vi "average position.vi"(1 "num lights":dbl, 2 "XYZ out":T1(array[cluster])) -> (0 "Lights pos":dbl[][](array[numeric]))   [LabVIEW 2011]
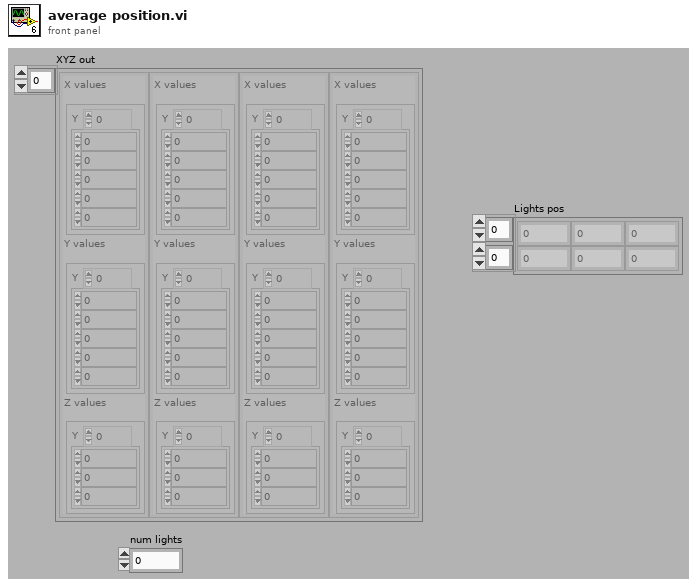
[diagram p1: front panel]
types:
  T1 = cluster{"X values":waveform(dbl), "Y values":waveform(dbl), "Z values":waveform(dbl)}[]
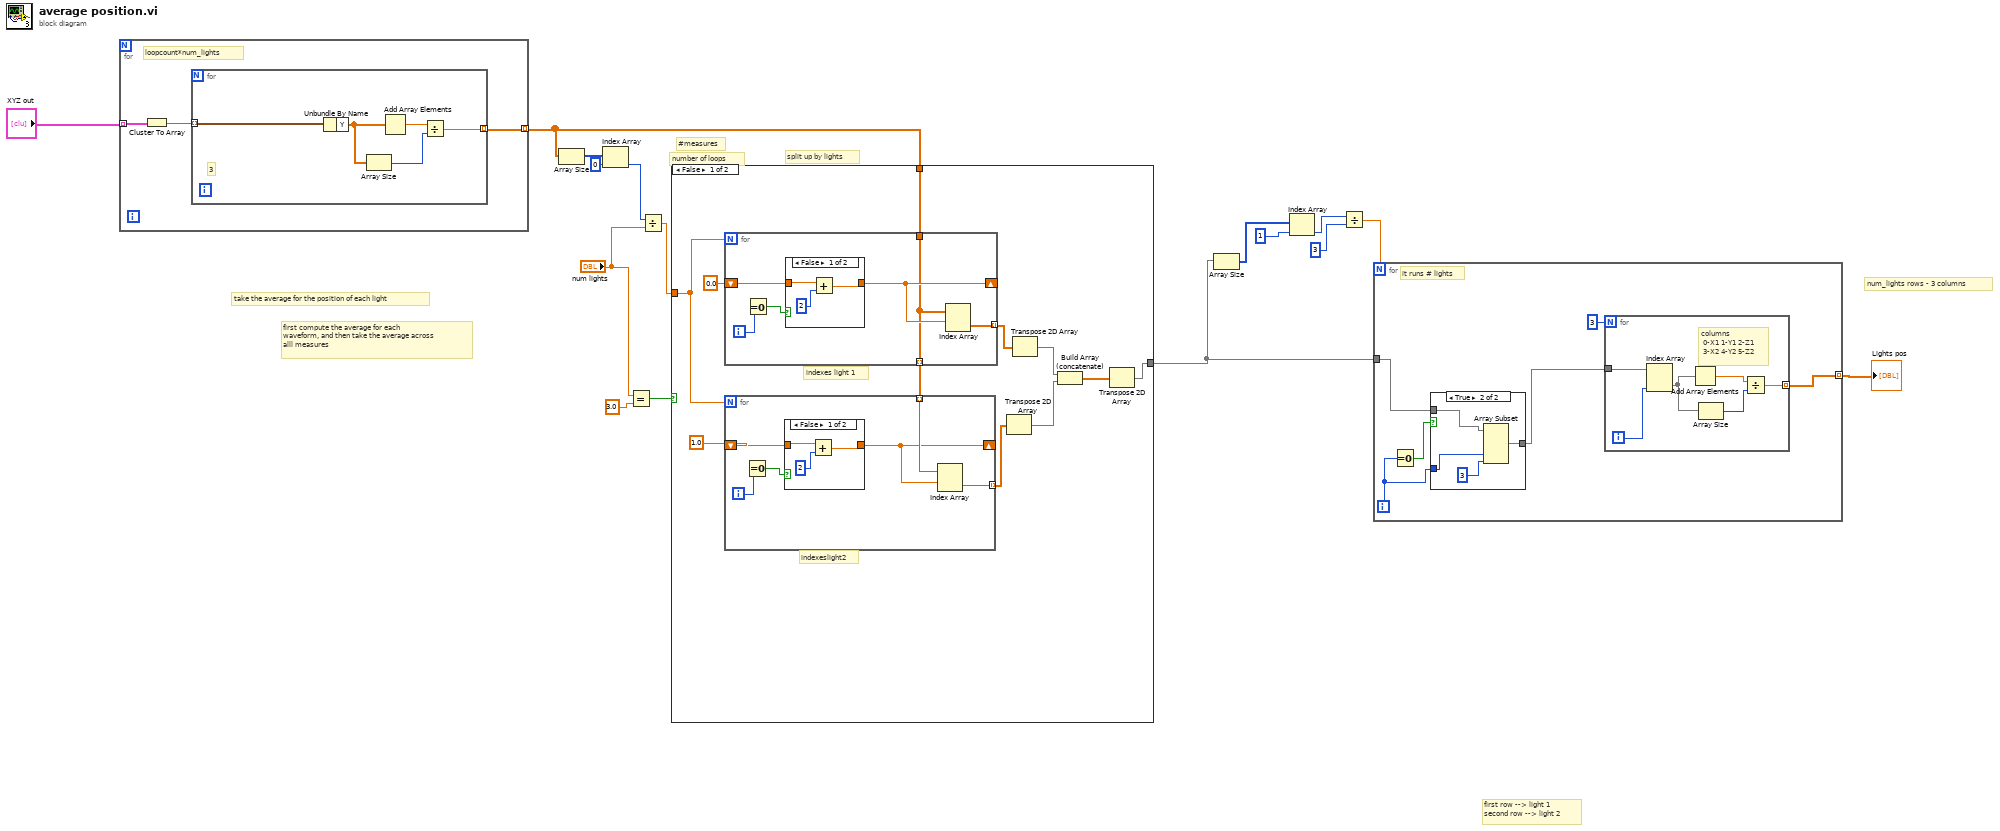
[diagram p0: block diagram]
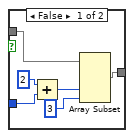
[diagram p2: hidden frame]
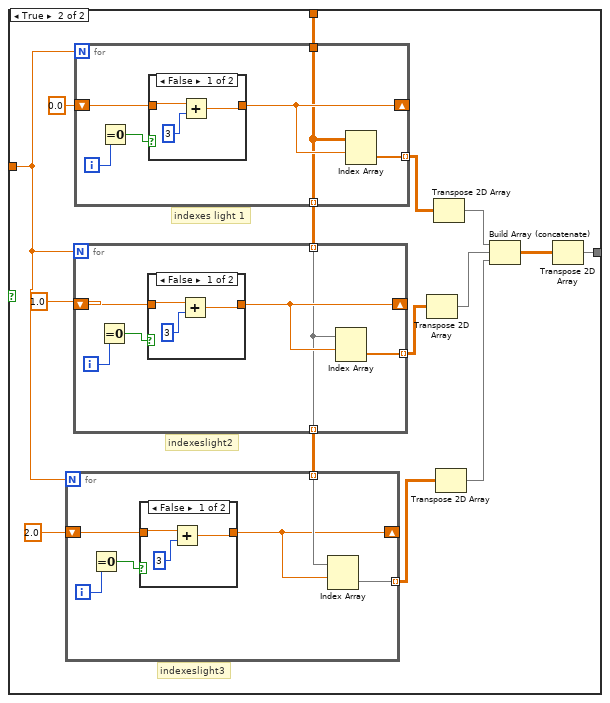
[diagram p5: hidden frame]
diagram:
  # "split up by lights"
  # "#measures"
  # "number of loops"
  # "num_lights rows - 3 columns"
  # "first compute the average for each \nwaveform, and then take the average across\nalll measures"
  # "first row --> light 1\nsecond row --> light 2"
  # "take the average for the position of each light"
  n1 = for {
    tunnel: [w19] -> w11 mode=indexing
    tunnel: "XYZ out" -> [w17] mode=indexing
    # "loopcount*num_lights"
    n2 = Cluster To Array(cluster=w17) -> (array=w18:waveform(dbl)[])
    n3 = for {
      tunnel: [w22] -> w19 mode=indexing
      tunnel: w18 -> [w21] mode=indexing
      # "3"
      n4 = Unbundle By Name(w21) -> ("Y"=w20:dbl[])
      n5 = Array Size(array=w20) -> (size(s)=w23:i32)
      n6 = Add Array Elements(numeric array=w20) -> (sum=w24:dbl)
      n7 = Divide(x=w24, y=w23) -> (x/y=w22:dbl)
    }
  }
  n8 = Array Size(array=w11) -> (size(s)=w15:i32[])
  n9 = Index Array(array=w15, index=0) -> (element=w13:i32)
  n10 = Equal?(x="num lights", y=3.0) -> (x = y?=w8:bool)
  n11 = Divide(x=w13, y="num lights") -> (x/y=w12:dbl)
  n12 = case shown="False" w8 {
    tunnel: w12 -> [w33 w65]
    tunnel: w11 -> [w32 w67]
    tunnel: [w25 w56] -> w2
    frame False {
      # "indexeslight2"
      # "indexes light 1"
      n13 = for {
        N: w33 -> [_]
        shift-right: [w48] -> _
        shift-left: 0.0 -> [w49]
        tunnel: w32 -> [w46]
        tunnel: [w47] -> w27 mode=indexing
        tunnel: [w46] -> w31 mode=indexing
        i -> [w51]
        n14 = Equal To 0?(x=w51) -> (x = 0?=w50:bool)
        n15 = case shown="False" w50 {
          tunnel: w49 -> [w54 w55]
          tunnel: [w52 w55] -> w48
          frame False {
            n16 = Add(x=w54, y=2) -> (x+y=w52:dbl)
          }
          frame True {
          }
        }
        n17 = Index Array(array=w46, index (row)=w48) -> (element=w47:dbl[])  [unwired: 1 in]
      }
      n18 = for {
        N: w33 -> [_]
        shift-right: [w37] -> _
        shift-left: 1.0 -> [w39]
        tunnel: w31 -> [w38] mode=indexing
        tunnel: [w36] -> w26 mode=indexing
        i -> [w41]
        n19 = Equal To 0?(x=w41) -> (x = 0?=w40:bool)
        n20 = case shown="False" w40 {
          tunnel: w39 -> [w44 w45]
          tunnel: [w42 w45] -> w37
          frame False {
            n21 = Add(x=w44, y=2) -> (x+y=w42:dbl)
          }
          frame True {
          }
        }
        n22 = Index Array(array=w38, index (row)=w37) -> (element=w36:dbl[])  [unwired: 1 in]
      }
      n23 = Transpose 2D Array(2D array=w26) -> (transposed array=w28:dbl[][])
      n24 = Transpose 2D Array(2D array=w27) -> (transposed array=w29:dbl[][])
      n25 = Build Array (concatenate)(w29, w28) -> (w30:dbl[][])
      n26 = Transpose 2D Array(2D array=w30) -> (transposed array=w25:dbl[][])
    }
    frame True {
      # "indexeslight3"
      # "indexeslight2"
      # "indexes light 1"
      n27 = for {
        N: w65 -> [_]
        shift-right: [w93] -> _
        shift-left: 0.0 -> [w94]
        tunnel: w67 -> [w91]
        tunnel: [w92] -> w60 mode=indexing
        tunnel: [w91] -> w68 mode=indexing
        i -> [w96]
        n28 = Equal To 0?(x=w96) -> (x = 0?=w95:bool)
        n29 = case shown="False" w95 {
          tunnel: w94 -> [w99 w100]
          tunnel: [w97 w100] -> w93
          frame False {
            n30 = Add(x=w99, y=3) -> (x+y=w97:dbl)
          }
          frame True {
          }
        }
        n31 = Index Array(array=w91, index (row)=w93) -> (element=w92:dbl[])  [unwired: 1 in]
      }
      n32 = for {
        N: w65 -> [_]
        shift-right: [w83] -> _
        shift-left: 1.0 -> [w84]
        tunnel: w68 -> [w81] mode=indexing
        tunnel: [w82] -> w59 mode=indexing
        tunnel: [w81] -> w66 mode=indexing
        i -> [w86]
        n33 = Equal To 0?(x=w86) -> (x = 0?=w85:bool)
        n34 = case shown="False" w85 {
          tunnel: w84 -> [w89 w90]
          tunnel: [w87 w90] -> w83
          frame False {
            n35 = Add(x=w89, y=3) -> (x+y=w87:dbl)
          }
          frame True {
          }
        }
        n36 = Index Array(array=w81, index (row)=w83) -> (element=w82:dbl[])  [unwired: 1 in]
      }
      n37 = for {
        N: w65 -> [_]
        shift-right: [w72] -> _
        shift-left: 2.0 -> [w74]
        tunnel: w66 -> [w73] mode=indexing
        tunnel: [w71] -> w58 mode=indexing
        i -> [w76]
        n38 = Equal To 0?(x=w76) -> (x = 0?=w75:bool)
        n39 = case shown="False" w75 {
          tunnel: w74 -> [w79 w80]
          tunnel: [w77 w80] -> w72
          frame False {
            n40 = Add(x=w79, y=3) -> (x+y=w77:dbl)
          }
          frame True {
          }
        }
        n41 = Index Array(array=w73, index (row)=w72) -> (element=w71:dbl[])  [unwired: 1 in]
      }
      n42 = Transpose 2D Array(2D array=w59) -> (transposed array=w63:dbl[][])
      n43 = Transpose 2D Array(2D array=w60) -> (transposed array=w62:dbl[][])
      n44 = Transpose 2D Array(2D array=w58) -> (transposed array=w57:dbl[][])
      n45 = Build Array (concatenate)(w62, w63, w57) -> (w61:dbl[][])
      n46 = Transpose 2D Array(2D array=w61) -> (transposed array=w56:dbl[][])
    }
  }
  n47 = Array Size(array=w2) -> (size(s)=w6:i32[])
  n48 = Index Array(array=w6, index=1) -> (element=w3:i32)
  n49 = Divide(x=w3, y=3) -> (x/y=w5:dbl)
  n50 = for {
    N: w5 -> [_]
    tunnel: w2 -> [w105]
    tunnel: [w106] -> w1 mode=indexing
    i -> [w103]
    # "it runs # lights"
    n51 = Equal To 0?(x=w103) -> (x = 0?=w104:bool)
    n52 = case shown="True" w104 {
      tunnel: w105 -> [w112 w116]
      tunnel: w103 -> [w111 w113]
      tunnel: [w109 w115] -> w102
      frame False {
        n53 = Add(x=2, y=w111) -> (x+y=w108:i32)
        n54 = Array Subset(array=w112, index (col)=w108, length (col)=3 ("length")) -> (w109:dbl[][])  [unwired: 2 in]
      }
      frame True {
        n55 = Array Subset(array=w116, index (col)=w113, length (col)=3 ("length")) -> (w115:dbl[][])  [unwired: 2 in]
      }
    }
    n56 = for {
      N: 3 -> [_]
      tunnel: w102 -> [w122]
      tunnel: [w117] -> w106 mode=indexing
      i -> [w119]
      # "columns\n 0-X1 1-Y1 2-Z1\n 3-X2 4-Y2 5-Z2"
      n57 = Index Array(array=w122, index (col)=w119) -> (element=w118:dbl[])  [unwired: 1 in]
      n58 = Add Array Elements(numeric array=w118) -> (sum=w120:dbl)
      n59 = Array Size(array=w118) -> (size(s)=w121:i32)
      n60 = Divide(x=w120, y=w121) -> (x/y=w117:dbl)
    }
  }
  "Lights pos" <- w1
